vi "Get All Deployed Stimulus Profile Sessions.vi"(8 "error in (no error)":errorcluster, 9 "Gateway IP Address (\"\": localhost)":string) -> (0 "error out":errorcluster, 3 "Deployed Session IDs":T1[](array[typedef]))   [LabVIEW 2020, in "NI_VS Sequence Execution Interface.lvlib"]
doc: "Queries the VeriStand Gateway and returns a list of all currently deployed stimulus profile sessions."
uses:
  <vilib>/NI VeriStand/Execution/SequenceExecutionInterface/NI_VS Sequence Execution Interface.lvlib
  <vilib>/NI VeriStand/Execution/SequenceExecutionInterface/Deployed Session Info.ctl
  <vilib>/NI VeriStand/Execution/SequenceExecutionInterface/Deployed Sequence Info.ctl
  <vilib>/NI VeriStand/Execution/SequenceExecutionInterface/Sequence Execution State.ctl
  NationalInstruments.VeriStand.ClientAPI
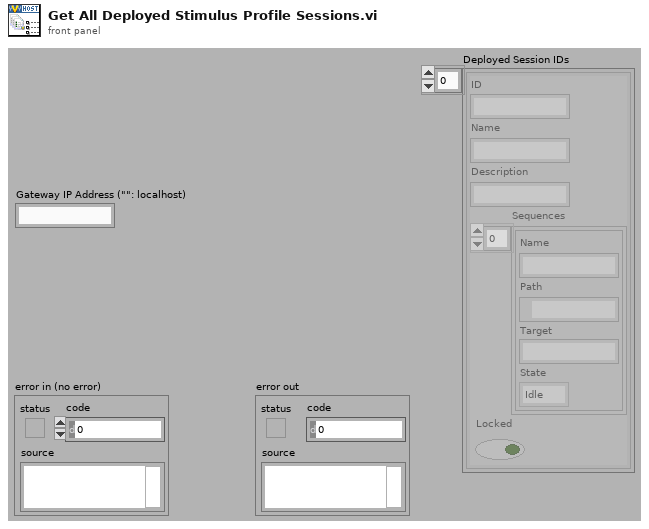
[diagram p1: front panel]
types:
  T1 = typedef "NI_VS Sequence Execution Interface.lvlib/Deployed Session Info.ctl" = cluster{"ID":string, "Name":string, "Description":string, "Sequences":T2[], "Locked":bool}
  T2 = typedef "NI_VS Sequence Execution Interface.lvlib/Deployed Sequence Info.ctl" = cluster{"Name":string, "Path":path, "Target":string, "State":T3}
  T3 = typedef "NI_VS Sequence Execution Interface.lvlib/Sequence Execution State.ctl" = enum16{"Idle", "Running", "SingleStepping", "Paused", "Stopped"}
  T4 = typedef "NI_VS Sequence Execution Interface.lvlib/Stimulus Profile Session Ref.ctl" = refnum<k24>
  T5 = typedef "NI_VS Sequence Execution Interface.lvlib/Sequence Call Ref.ctl" = refnum<k24>
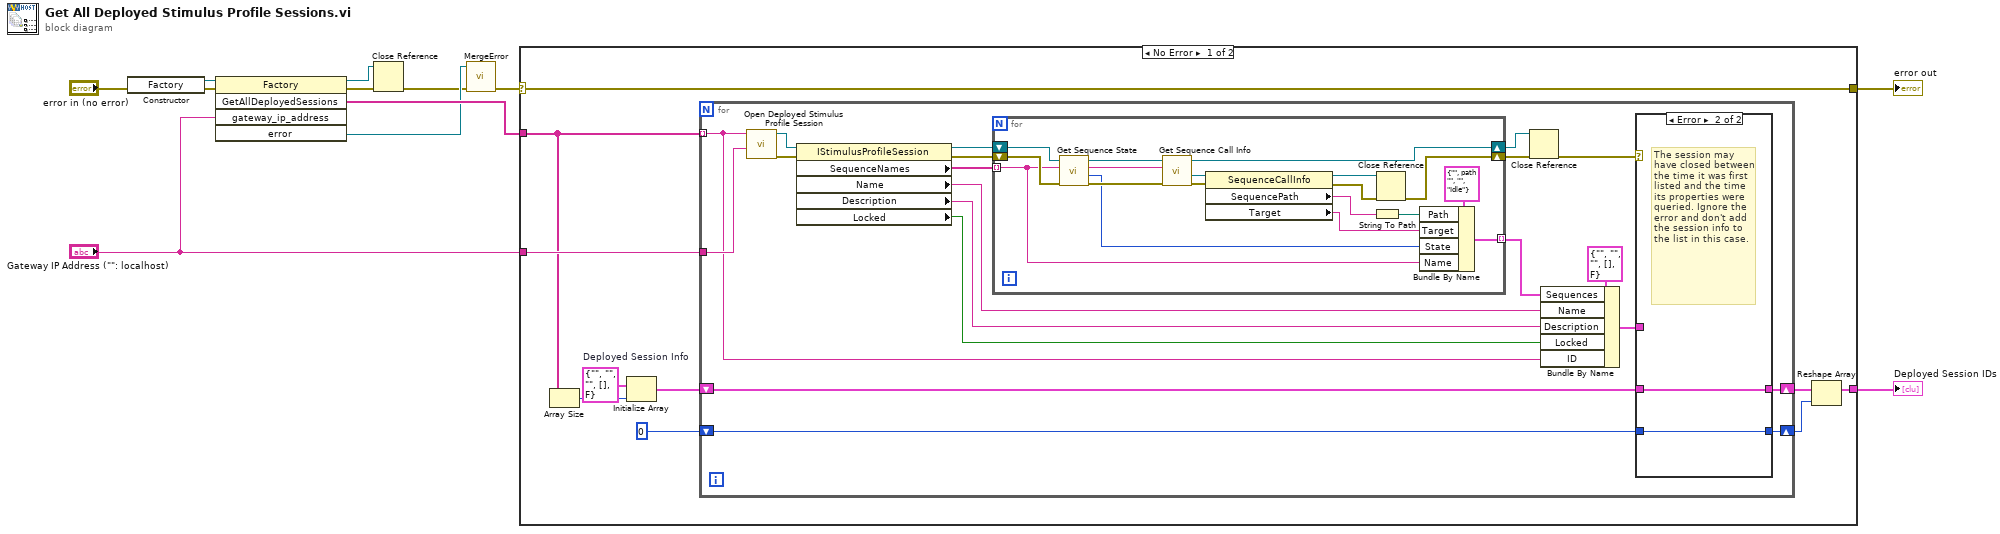
[diagram p0: block diagram]
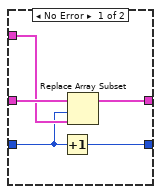
[diagram p2: hidden frame]
diagram:
  n1 = constructor class="Factory"(error in="error in (no error)") -> (reference out=w8:refnum<k24>, error out=w7:errorcluster)  [unwired: 2 in, 1 out]
  n2 = invoke class="Factory" method="GetAllDeployedSessions"(reference=w8, error in=w7, "gateway_ip_address"="Gateway IP Address (\"\": localhost)") -> (reference out=w1:refnum<k24>, error out=w3:errorcluster, "GetAllDeployedSessions"=w5:string[], "error"=w4:refnum<k24>)  [unwired: 2 in, 1 out]
  n3 = Close Reference(reference=w1, error in (no error)=w3) -> (error out=w2:errorcluster)
  n4 = call <vilib>:"MergeError.vi"("error in (no error)"=w2, "Error"=w4) -> ("error out"=w9:errorcluster)  [unwired: 9 out]
  n5 = case shown="No Error" w9 {
    selector: w9 -> [w21 w68]
    tunnel: w5 -> [w20 _]
    tunnel: "Gateway IP Address (\"\": localhost)" -> [w22 _]
    tunnel: [w21 w68] -> w10
    tunnel: [w13 _] -> w11
    frame No Error {
      w19 = T1 {"ID"="", "Name"="", "Description"="", "Sequences"=[], "Locked"=FALSE}  # Deployed Session Info
      n6 = Array Size(array=w20) -> (size(s)=w18:i32)
      n7 = Initialize Array(w19, w18) -> (w17:T1[])
      n8 = for {
        tunnel: w22 -> [w42]
        tunnel: w20 -> [w37] mode=indexing
        shift-right: [w27] -> w15
        shift-left: w17 -> [w26]
        shift-right: [w24] -> w14
        shift-left: 0 -> [w23]
        n9 = call <vilib>:"Open Deployed Stimulus Profile Session.vi"("Gateway IP Address (\"\": localhost)"=w42, "Deployed Session ID"=w37) -> ("error out"=w41:errorcluster, "Session Ref"=w40:T4)  [unwired: 8 in]
        n10 = property class="IStimulusProfileSession"(reference=w40, error in=w41) -> (reference out=w34:T4, error out=w35:errorcluster, "SequenceNames"=w31:string[], "Name"=w32:string, "Description"=w39:string, "Locked"=w38:bool)
        n11 = for {
          shift-right: [w54] -> w29
          shift-left: w35 -> [w59]
          shift-right: [w53] -> w33
          shift-left: w34 -> [w58]
          tunnel: w31 -> [w52] mode=indexing
          tunnel: [w64] -> w30 mode=indexing
          n12 = call <vilib>:"Get Sequence State.vi"("error in (no error)"=w59, "Sequence Name"=w52, "Session Ref in"=w58) -> ("error out"=w67:errorcluster, "State"=w56:T3, "Sequence Name out"=w50:string, "Session Ref out"=w51:T4)  [unwired: 5 in]
          n13 = call <vilib>:"Get Sequence Call Info.vi"("error in (no error)"=w67, "Sequence Name"=w50, "Session Ref in"=w51) -> ("error out"=w55:errorcluster, "Sequence Call Ref"=w57:T5, "Session Ref out"=w53:T4)  [unwired: 5 in, 1 out]
          n14 = property class="SequenceCallInfo"(reference=w57, error in=w55) -> (reference out=w60:T5, error out=w66:errorcluster, "SequencePath"=w63:string, "Target"=w61:string)
          n15 = String To Path(string=w63) -> (path=w62:path)
          n16 = Close Reference(reference=w60, error in (no error)=w66) -> (error out=w54:errorcluster)
          n17 = Bundle By Name(cluster=T2 {"Name"="", "Path"=path "", "Target"="", "State"=enum."Idle"} ("Deployed Sequence Info"), "Path"=w62, "Target"=w61, "State"=w56, "Name"=w52) -> (w64:T2)
        }
        n18 = Close Reference(reference=w33, error in (no error)=w29) -> (error out=w25:errorcluster)
        n19 = Bundle By Name(cluster=T1 {"ID"="", "Name"="", "Description"="", "Sequences"=[], "Locked"=FALSE} ("Deployed Session Info"), "Sequences"=w30, "Name"=w32, "Description"=w39, "Locked"=w38, "ID"=w37) -> (w28:T1)
        n20 = case shown="Error" w25 {
          tunnel: w28 -> [w45 _]
          tunnel: [w46 w49] -> w27
          tunnel: w26 -> [w47 w49]
          tunnel: [w43 w48] -> w24
          tunnel: w23 -> [w44 w48]
          frame No Error {
            n21 = Increment(x=w44) -> (x+1=w43:i32)
            n22 = Replace Array Subset(array=w47, new element=w45, index=w44) -> (w46:T1[])
          }
          frame Error {
            # "The session may have closed between the time it was first listed and the time its properties were queried. Ignore the error and don't add the session info to the list in this case."
          }
        }
      }
      n23 = Reshape Array(w15, w14) -> (w13:T1[])
    }
    frame Error {
    }
  }
  "error out" <- w10
  "Deployed Session IDs" <- w11
